vi "U32 reverse bytes.vi"(1 "U32 in":u32) -> (0 "U32 out":u32)   [LabVIEW 2013]
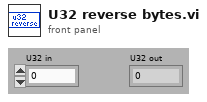
[diagram p1: front panel]
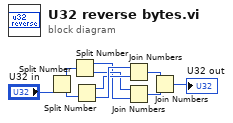
[diagram p0: block diagram]
diagram:
  n1 = Split Number(x="U32 in") -> (hi(x)=w2:u16, lo(x)=w3:u16)
  n2 = Split Number(x=w2) -> (hi(x)=w4:u8, lo(x)=w5:u8)
  n3 = Split Number(x=w3) -> (hi(x)=w6:u8, lo(x)=w7:u8)
  n4 = Join Numbers(hi=w7, lo=w6) -> ((hi.lo)=w8:u16)
  n5 = Join Numbers(hi=w5, lo=w4) -> ((hi.lo)=w9:u16)
  n6 = Join Numbers(hi=w8, lo=w9) -> ((hi.lo)=→"U32 out":u32)
